vi "calcTRABS-SD.vi"(2 "II channel seq":T1, 3 "I channel seq":T1) -> (0 "TRans shifted":dbl[][](array[numeric]), 1 "TRanS multiple measurements":dbl[][](array[numeric]))   [LabVIEW 2015]
uses:
  controls/data-cluster.ctl
panel:
  # "Transmission: on fait le log après la moyenne.\n\nCe VI comporte une entrée Dark: dark shutter fermé. La laisser à 0 \nce dark doit être retiré à toute les données, puis on doit faire le meme calcul avec le reste de Idark -dark à la place de Idark.s"
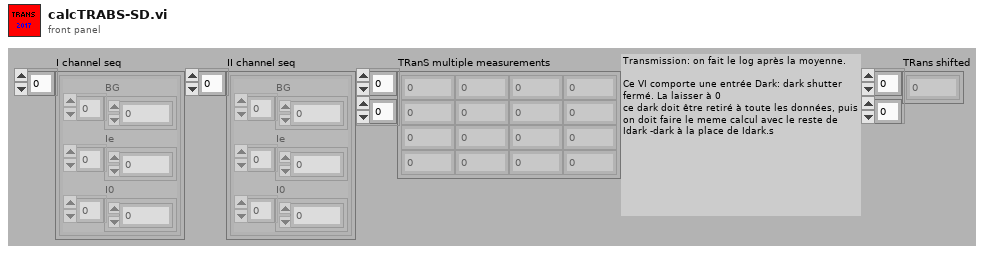
[diagram p1: front panel]
types:
  T1 = typedef "data-cluster.ctl" = cluster{"BG":i32[], "Ie":i32[], "I0":i32[]}[]
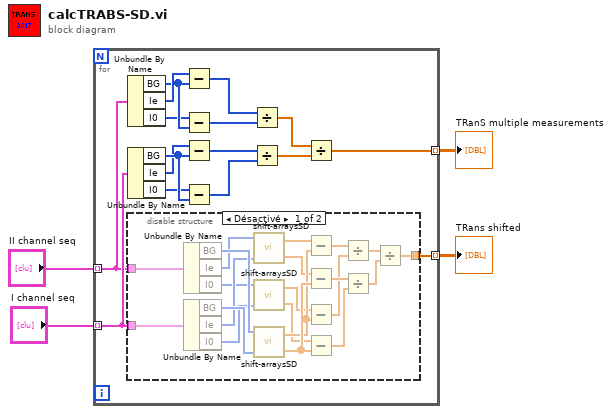
[diagram p0: block diagram]
diagram:
  n1 = for {
    tunnel: "I channel seq" -> [w13] mode=indexing
    tunnel: "II channel seq" -> [w12] mode=indexing
    tunnel: [w14] -> w4 mode=indexing
    tunnel: [w5] -> w1 mode=indexing
    n2 = Unbundle By Name(w12) -> ("BG"=w10:i32[], "Ie"=w11:i32[], "I0"=w9:i32[])
    n3 = Unbundle By Name(w13) -> ("BG"=w8:i32[], "Ie"=w7:i32[], "I0"=w6:i32[])
    n4 = disable-structure shown="Désactivé" {
      disable-tunnel: w13 -> [w41 _]
      disable-tunnel: w12 -> [w40 _]
      disable-tunnel: [w33 _] -> w5
      frame Disabled {
        n5 = Unbundle By Name(w40) -> ("BG"=w32:i32[], "Ie"=w28:i32[], "I0"=w24:i32[])
        n6 = Unbundle By Name(w41) -> ("BG"=w31:i32[], "Ie"=w27:i32[], "I0"=w23:i32[])
        n7 = call "shift-arraysSD.vi"("in2"=w27, "in1"=w28) -> ("out2"=w25:dbl[], "out1"=w26:dbl[])  [unwired: 1 in]
        n8 = call "shift-arraysSD.vi"("in2"=w23, "in1"=w24) -> ("out2"=w21:dbl[], "out1"=w22:dbl[])  [unwired: 1 in]
        n9 = call "shift-arraysSD.vi"("in2"=w31, "in1"=w32) -> ("out2"=w30:dbl[], "out1"=w29:dbl[])  [unwired: 1 in]
        n10 = Subtract(x=w26, y=w29) -> (x-y=w34:dbl[])
        n11 = Subtract(x=w25, y=w30) -> (x-y=w36:dbl[])
        n12 = Subtract(x=w22, y=w29) -> (x-y=w35:dbl[])
        n13 = Subtract(x=w21, y=w30) -> (x-y=w37:dbl[])
        n14 = Divide(x=w34, y=w35) -> (x/y=w38:dbl[])
        n15 = Divide(x=w36, y=w37) -> (x/y=w39:dbl[])
        n16 = Divide(x=w38, y=w39) -> (x/y=w33:dbl[])
      }
      frame Enabled {
      }
    }
    n17 = Subtract(x=w11, y=w10) -> (x-y=w20:i32[])
    n18 = Subtract(x=w9, y=w10) -> (x-y=w19:i32[])
    n19 = Subtract(x=w7, y=w8) -> (x-y=w18:i32[])
    n20 = Subtract(x=w6, y=w8) -> (x-y=w17:i32[])
    n21 = Divide(x=w20, y=w19) -> (x/y=w16:dbl[])
    n22 = Divide(x=w18, y=w17) -> (x/y=w15:dbl[])
    n23 = Divide(x=w16, y=w15) -> (x/y=w14:dbl[])
  }
  "TRanS multiple measurements" <- w4
  "TRans shifted" <- w1
